vi "Compute Drivetrain Values.vi"(0 "Motor Type":T3=enum."Neo", 1 "Gear Ratio (out/in)":dbl=0.05 step=0.01, 2 "Robot Characterization":T1={"Total Mass"=68.0388555, "Wheel Friction"=1.0, "Wheel Diameter"=0.15239999999999998}, 3 "Loop Time":dbl[unit] format="%#_13g") -> (7 "Array":T4(array[cluster]))   [LabVIEW 2019]
uses:
  <vilib>/addons/control/pid/NI_PID_pid.lvlib
  <vilib>/addons/control/pid/pid.llb/PID (DBL).vi
  Motor Type.ctl
  Modeling/Battery Coefficients.ctl
panel:
  in  "Include Droop":bool=TRUE
  in  "Current Limit":dbl[unit]=50.0 format="%#_13g"
  in  "Torque Efficiency":dbl=0.8 format="%#_13g"
  in  "Motor Count":dbl=6.0 format="%#_13g"
  in  "Breaker":dbl[unit]=30.0
  in  "Battery Characterization":T2={"Battery Voltage"=12.9, "Internal Resistance"=0.015, "Battery Capacity"=64800.0, "Battery Temp"=75.0, "Battery Weight"=5.4431084400000005, "State of Charge %"=12.0} {"State of Charge %" format="%#_13g"; "Battery Weight" format="%#_13g"; "Battery Temp" format="%#_13g"; "Battery Capacity" format="%#_13g"; "Internal Resistance" format="%#_13g"; "Battery Voltage" format="%#_13g"}
  in  "stop":bool
  in  "Initial RPM":dbl
  out "Waveform Chart":dbl[unit](graph)
  out "slip":bool
  in  "Timestep":dbl[unit]=0.001 format="%#_3p"
  out "secs":dbl
  out "Brownout":bool
  in  "Control":enum32{"Manual", "! !", "PID"}(tab)
  in  "Vbus %":dbl(slide)=27.27272727272728 scale=-100.0..100.0
  in  "When below":dbl[unit]=9.0
  in  "When Above":dbl[unit]
  in  "PID gains":T5={"proportional gain (Kc)"=1.9999999999999987, "integral time (Ti, min)"=0.0, "derivative time (Td, min)"=0.0} {"derivative time (Td, min)" format="%.3f"; "integral time (Ti, min)" format="%.3f"; "proportional gain (Kc)" format="%.3f"}
  in  "Setpoint RPM":dbl(slide)=4000.0 scale=-5820.0..5820.0
  out "Chart":T6(graph)
  # "Motor Information"
  # "Robot Information"
  # "Battery Information"
  # "Simulation Information"
  # "Simulation"
  # "RPM\n\nMotor V\n\nCurrent\n\nBatt V\n\nSpeed fps\n\nDistance ft\n\nSlip"
  # "Missing Features:\nAdd breaker state"
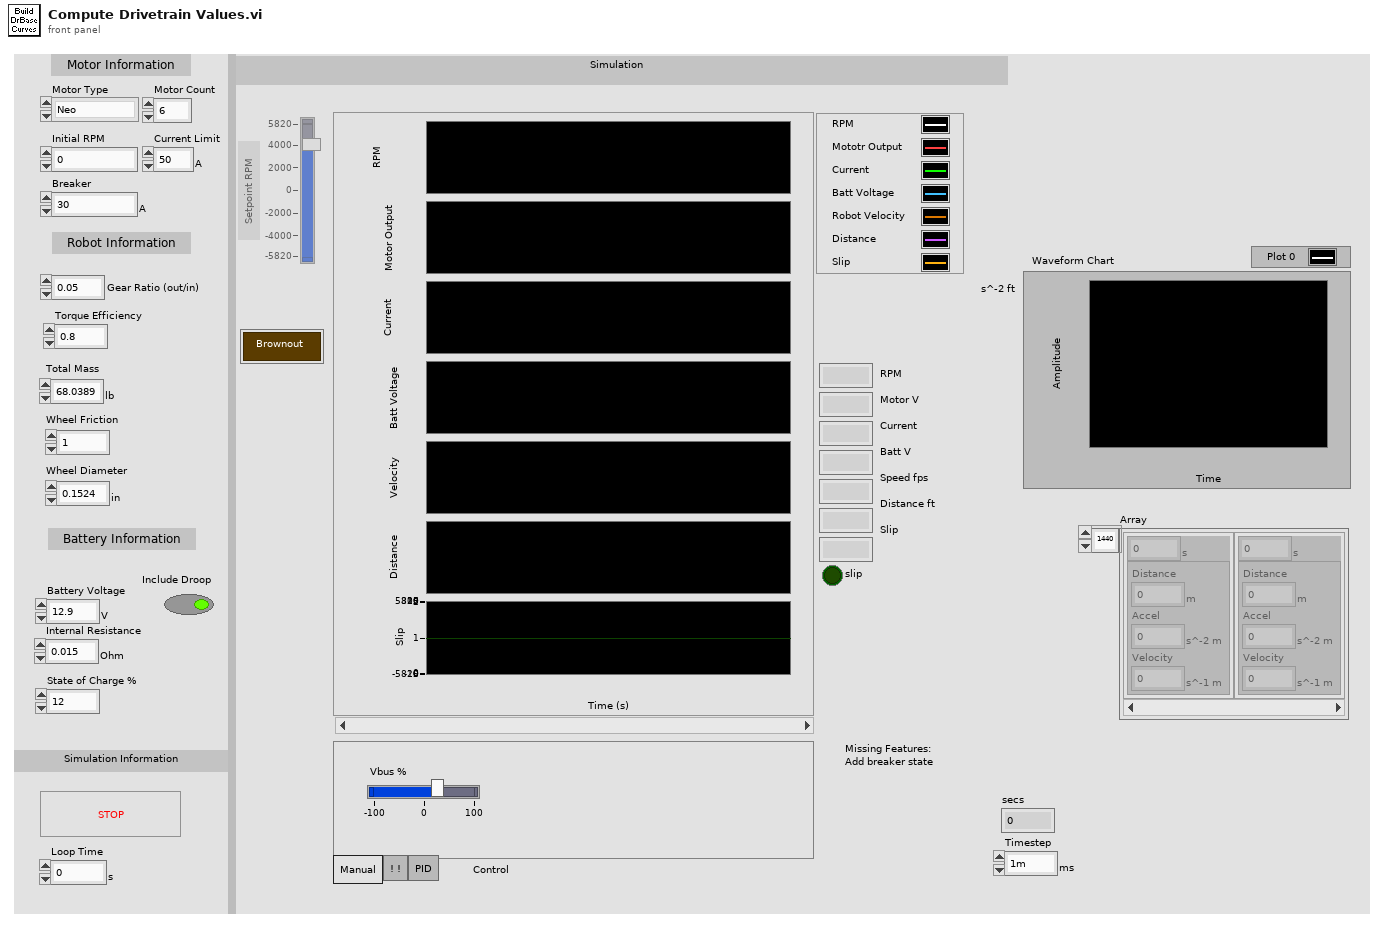
[diagram p1: front panel]
types:
  T1 = cluster{"Total Mass":dbl[unit], "Wheel Friction":dbl, "Wheel Diameter":dbl[unit]}
  T2 = typedef "Battery Coefficients.ctl" = cluster{"Battery Voltage":dbl[unit], "Internal Resistance":dbl[unit], "Battery Capacity":dbl[unit], "Battery Temp":dbl[unit], "Battery Weight":dbl[unit], "State of Charge %":dbl}
  T3 = typedef "Motor Type.ctl" = enum16{"Custom", "775 pro", "CIM", "miniCIM", "Neo", "Neo 550", "Falcon 500"}
  T4 = cluster{dbl[unit], cluster{"Distance":dbl[unit], "Accel":dbl[unit], "Velocity":dbl[unit]}}[]
  T5 = cluster{"proportional gain (Kc)":dbl, "integral time (Ti, min)":dbl, "derivative time (Td, min)":dbl}
  T6 = cluster{"Initial RPM":dbl, "Motor Voltage":dbl[unit], dbl[unit], "Battery Voltage":dbl[unit], "Current":dbl[unit], "Current":dbl[unit], i16}
  T7 = cluster{"Initial RPM":dbl, "When Above":dbl[unit], dbl[unit], "Battery Voltage":dbl[unit], dbl[unit], dbl[unit], i32}[]
  T8 = typedef "Motor Operating Values.ctl" = cluster{"Kv":dbl[unit], "R":dbl[unit], "Kt":dbl[unit], "Breaker Size":dbl[unit]}
  T9 = enum8{"Enabled", "Disabled", "Disabled and Grayed Out"}
  T10 = cluster{"Distance":dbl[unit], "Robot Accel":dbl[unit], "Velocity":dbl[unit]}
  T11 = cluster{"Initial RPM":dbl, "Motor Voltage":dbl[unit], dbl[unit], "Battery Voltage":dbl[unit], "Velocity":dbl[unit], "Distance":dbl[unit], i16}
  T12 = cluster{dbl[unit], cluster{"Distance":dbl[unit], "Robot Accel":dbl[unit], "Velocity":dbl[unit]}}
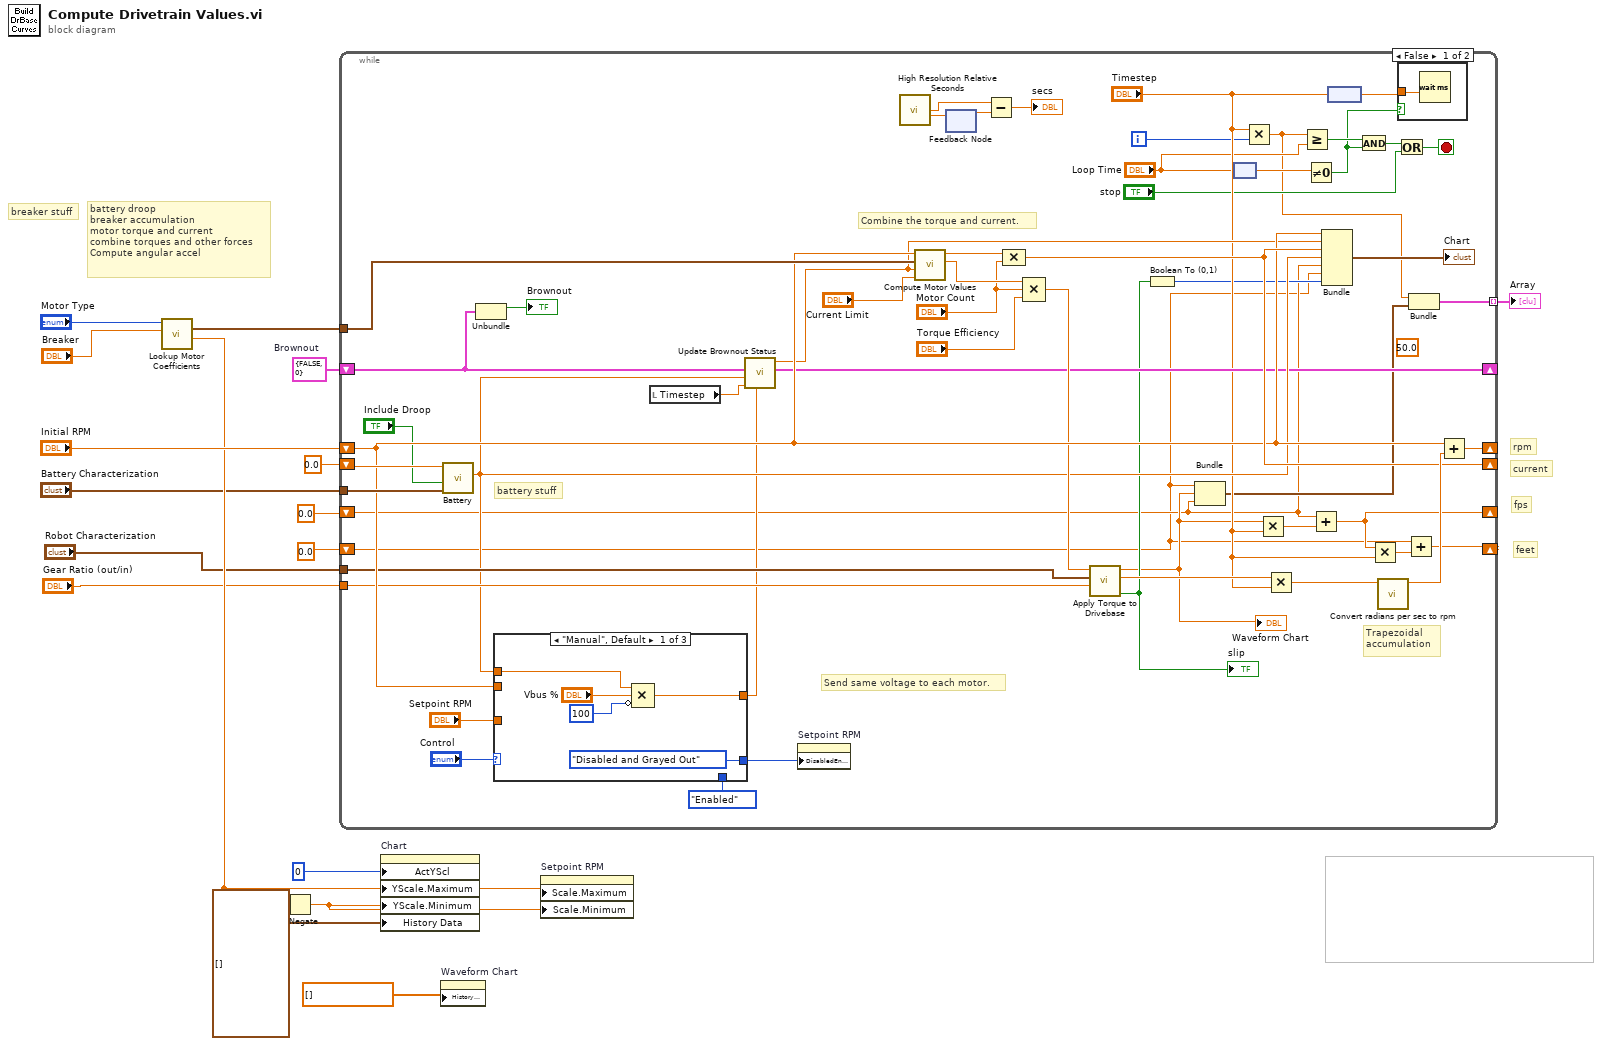
[diagram p0: block diagram]
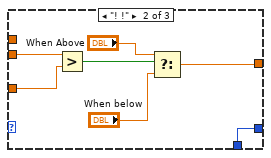
[diagram p3: hidden frame]
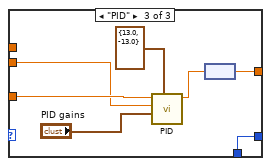
[diagram p4: hidden frame]
diagram:
  w3 = cluster{bool, i32} {FALSE, 0}  # Brownout
  # "breaker stuff"
  # "feet"
  # "fps"
  # "current"
  # "rpm"
  # "battery droop\nbreaker accumulation\nmotor torque and current\ncombine torques and other forces\nCompute angular accel"
  n1 = call "Lookup Motor Coefficients.vi"("Breaker Size"="Breaker", "Motor Type"="Motor Type") -> ("Free Speed"=w12:dbl, "Motor Model Values"=w16:T8)  [unwired: 6 in, 2 out]
  n2 = Negate(x=w12) -> (-x=w11:dbl)
  n3 = while {
    tunnel: w16 -> [w61]
    shift-right: [w72] -> _
    shift-left: "Initial RPM" -> [w58]
    shift-right: [w60] -> _
    shift-left: dbl[unit] 0.0 ("Current") -> [w64]
    tunnel: "Battery Characterization" -> [w59]
    tunnel: "Robot Characterization" -> [w53]
    tunnel: "Gear Ratio (out/in)" -> [w52]
    shift-right: [w47] -> _
    shift-left: dbl[unit] 0.0 ("Velocity") -> [w19]
    shift-right: [w48] -> _
    shift-left: dbl[unit] 0.0 ("Distance") -> [w18]
    shift-right: [w44] -> _
    shift-left: w3 -> [w46]
    tunnel: [w25] -> w2 mode=indexing
    i -> [w34]
    stop <- w32 stop-if-true
    (unwired) 50.0
    # "Combine the torque and current."
    # "Trapezoidal\naccumulation"
    # "Send same voltage to each motor."
    # "battery stuff"
    n4 = call "Battery.vi"("Battery Characterization"=w59, "Include Droop"="Include Droop", "Current"=w64) -> ("Battery Voltage"=w45:dbl[unit])  [unwired: 8 in]
    n5 = Unbundle(w46) -> (→"Brownout":bool)  [unwired: 1 out]
    n6 = case shown="\"Manual\", Default" "Control" {
      tunnel: [w77 w82 w87] -> w43
      tunnel: w58 -> [_ w85 w90]
      tunnel: "Setpoint RPM" -> [_ w80 w91]
      tunnel: [T9."Disabled and Grayed Out" ("Disabled") w79 w86] -> w65
      tunnel: T9."Enabled" ("Disabled") -> [_ w79 w86]
      tunnel: w45 -> [w74 _ _]
      frame "Manual", Default {
        n7 = Compound Arithmetic op=MULTIPLY(w74, "Vbus %", invert 100) -> (w77:dbl[unit])
      }
      frame "! !" {
        n8 = Greater?(x=w85, y=w80) -> (0:w84:bool)
        n9 = Select(t="When Above", s=w84, f="When below") -> (s? t:f=w82:dbl[unit])
      }
      frame "PID" {
        n10 = call-poly <vilib>:"PID.vi"("output range"=cluster{"output high":dbl, "output low":dbl} {"output high"=13.0, "output low"=-13.0}, "PID gains"="PID gains", "process variable"=w90, "setpoint"=w91) -> ("output"=w88:dbl)  [unwired: 6 in, 1 out]
        n11 = node(w88) -> (w87:dbl[unit])
      }
    }
    n12 = local read "Timestep"() -> (w37:dbl[unit])
    n13 = call "Update Brownout Status.vi"("VBus"=w43, "Timestep"=w37, "Battery Voltage"=w45, "Brownout in"=w46) -> ("Brownout status"=w44:cluster{bool, u32}, "Motor Voltage"=w42:dbl[unit])  [unwired: 6 in]
    n14 = property on="Setpoint RPM" class="Slide (strict)"("DisabledEnum"=w65) -> ()  [unwired: 2 in, 2 out]
    n15 = call <vilib>:"High Resolution Relative Seconds.vi"() -> ("relative seconds"=w39:dbl)
    n16 = call "Compute Motor Values.vi"("Current Limit"="Current Limit", "Effective Motor Voltage"=w42, "Motor Model Values"=w61, "motor speed (rpm)"=w58) -> ("Motor Torque"=w62:dbl[unit], "Current"=w63:dbl[unit])  [unwired: 4 in, 2 out]
    n17 = feedback-in #1(w39) -> ()
    n18 = feedback #1() -> (w40:dbl)  [unwired: 1 in]
    n19 = Subtract(x=w39, y=w40) -> (x-y=→"secs":dbl)
    n20 = Compound Arithmetic op=MULTIPLY(w63, "Motor Count") -> (w60:dbl[unit])
    n21 = Compound Arithmetic op=MULTIPLY(w62, "Motor Count", "Torque Efficiency") -> (w54:dbl[unit])
    n22 = call "Apply Torque to Drivebase.vi"("Gear Ratio (out/in)"=w52, "Robot Characterization"=w53, "Motor Torque"=w54) -> ("slip"=w23:bool, "Motor Angular accel"=w51:dbl[unit], "Robot Accel"=w20:dbl[unit])  [unwired: 6 in]
    "slip" <- w23
    "Waveform Chart" <- w20
    n23 = Boolean To (0,1)(Boolean=w23) -> (0, 1=w22:i16)
    n24 = Bundle("Distance"=w18, "Robot Accel"=w20, "Velocity"=w19) -> (w21:T10)  [unwired: 1 in]
    n25 = node("Loop Time") -> (w30:dbl)
    n26 = Multiply(x="Timestep", y=w34) -> (x*y=w26:dbl[unit])
    n27 = Multiply(x=w20, y="Timestep") -> (x*y=w50:dbl[unit])
    n28 = Multiply(x=w51, y="Timestep") -> (x*y=w70:dbl[unit])
    n29 = Greater Or Equal?(x=w26, y="Loop Time") -> (x >= y?=w29:bool)
    n30 = Not Equal To 0?(x=w30) -> (x != 0?=w24:bool)
    n31 = Add(x=w19, y=w50) -> (x+y=w47:dbl[unit])
    n32 = Bundle("Initial RPM"=w58, "Motor Voltage"=w42, w60, "Battery Voltage"=w45, "Velocity"=w19, "Distance"=w18, w22) -> (→"Chart":T11)  [unwired: 1 in]
    n33 = node("Timestep") -> (w69:dbl)
    n34 = And(x=w29, y=w24) -> (x .and. y?=w28:bool)
    n35 = Multiply(x=w47, y="Timestep") -> (x*y=w49:dbl[unit])
    n36 = call "Convert radians per sec to rpm.vi"("speed in"=w70) -> ("speed out (rpm)"=w71:dbl)  [unwired: 10 in]
    n37 = Or(x=w28, y="stop") -> (x .or. y?=w32:bool)
    n38 = case shown="False" w24 {
      tunnel: w69 -> [w73 _]
      frame False {
        n39 = Wait (ms)(milliseconds to wait=w73) -> ()  [unwired: 1 out]
      }
      frame True {
      }
    }
    n40 = Add(x=w18, y=w49) -> (x+y=w48:dbl[unit])
    n41 = Bundle(w26, w21) -> (w25:T12)  [unwired: 1 in]
    n42 = Add(x=w58, y=w71) -> (x+y=w72:dbl)
  }
  "Array" <- w2
  n43 = property on="Chart" class="WFChart (strict)"("ActYScl"=0 ("Active Y Scale"), "YScale.Maximum"=w12, "YScale.Minimum"=w11, "History Data"=T7 []) -> ()  [unwired: 2 in, 2 out]
  n44 = property on="Waveform Chart" class="WFChart (strict)"("History Data"=dbl[unit][] []) -> ()  [unwired: 2 in, 2 out]
  n45 = property on="Setpoint RPM" class="Slide (strict)"("Scale.Maximum"=w12, "Scale.Minimum"=w11) -> ()  [unwired: 2 in, 2 out]
